vi "Weak AI Player.vi"(0 "Total Player number":i32, 1 "Current Player ID number":i32, 2 "queue output":refnum<queue>, 3 "queue input":refnum<queue>) -> ()   [LabVIEW 2021]
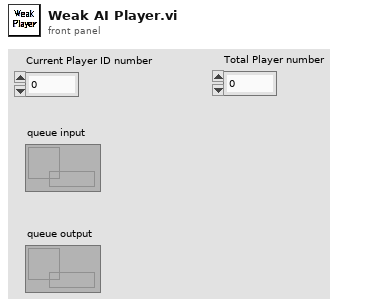
[diagram p1: front panel]
types:
  T1 = cluster{"X":dbl, "Y":dbl, "Object type":dbl, "Radius":dbl, "Width":dbl, "Height":dbl, "Theta":dbl, "HP":dbl, "R":dbl, "G":dbl, "B":dbl}[]
  T2 = cluster{"D1":dbl, "D2":dbl, "D3":dbl, "D4":dbl, "D5":dbl, "D6":dbl, "D7":dbl, "D8":dbl}
  T3 = cluster{"D1":bool, "D2":bool, "D3":bool, "D4":bool, "D5":bool, "D6":bool, "D7":bool, "D8":bool}
  T4 = cluster{"X":dbl, "Y":dbl, "Object type":dbl, "Radius":dbl, "Width":dbl, "Height":dbl, "Theta":dbl, "HP":dbl, "R":dbl, "G":dbl, "B":dbl}
  T5 = cluster{"Theta (toward that target)":dbl, "Distance (toward that target)":dbl, "Reachable":bool}
  T6 = cluster{dbl, dbl, "y":dbl, "y":dbl, "y":dbl, "y":dbl}
  T7 = cluster{dbl, dbl, "Theta (toward that target)":dbl, "f":dbl}
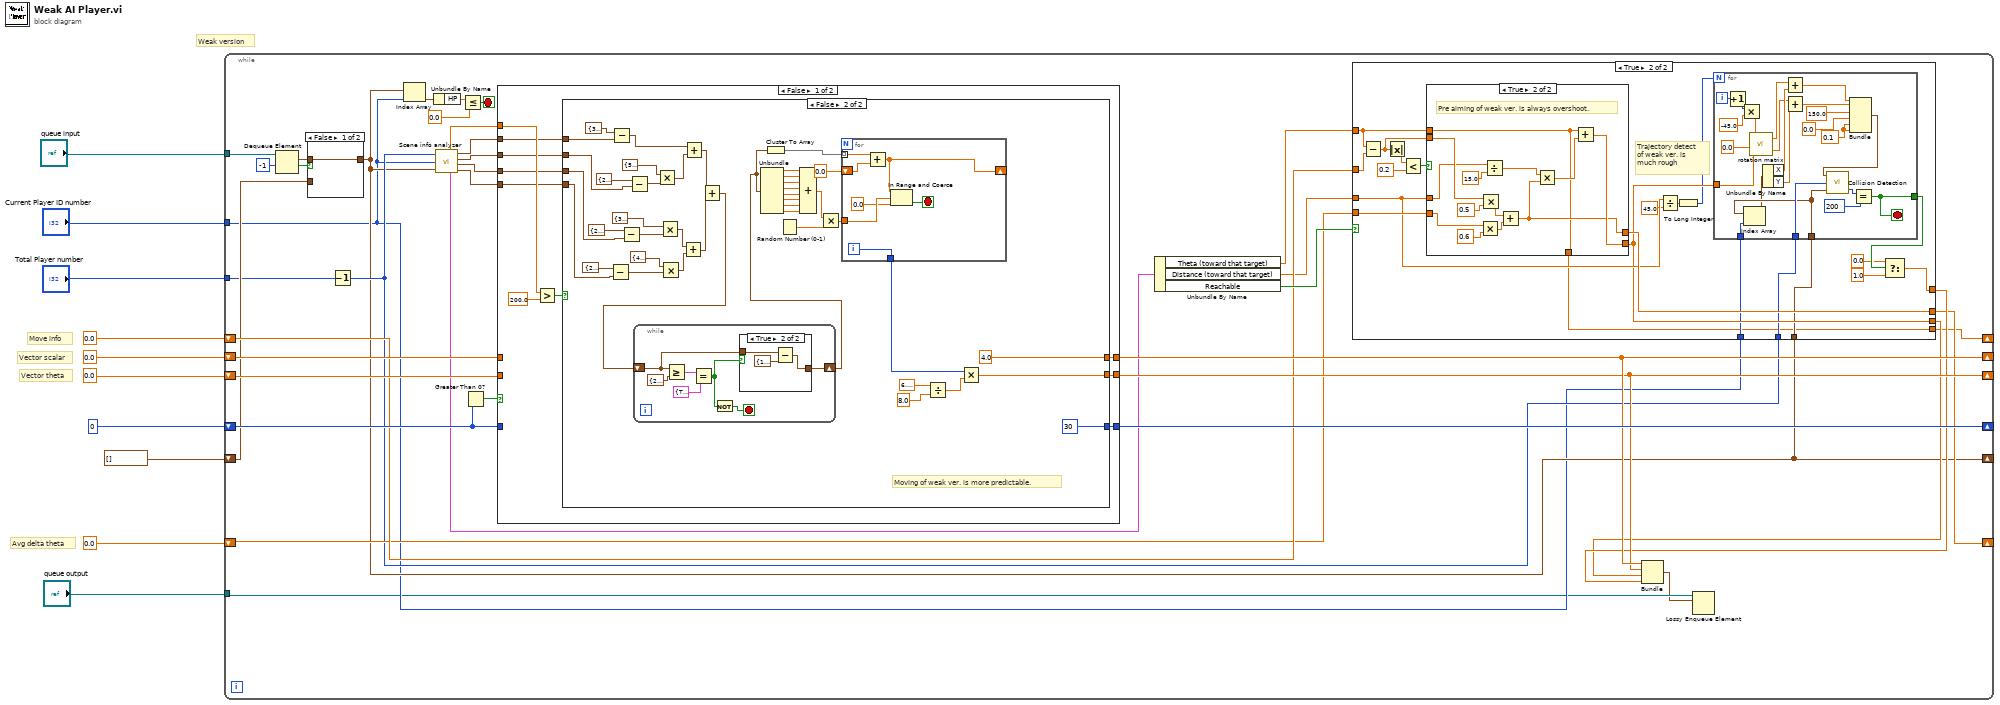
[diagram p0: block diagram]
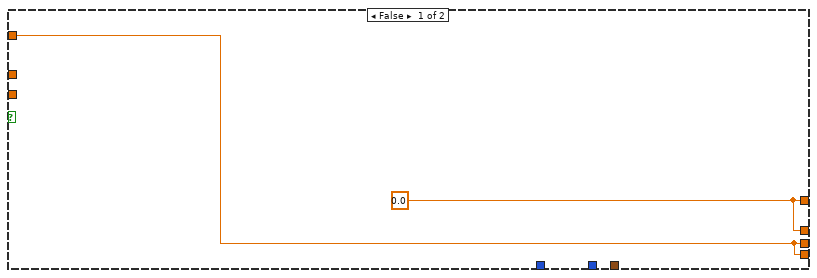
[diagram p3: hidden frame]
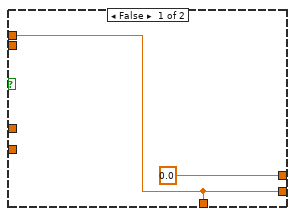
[diagram p4: hidden frame]
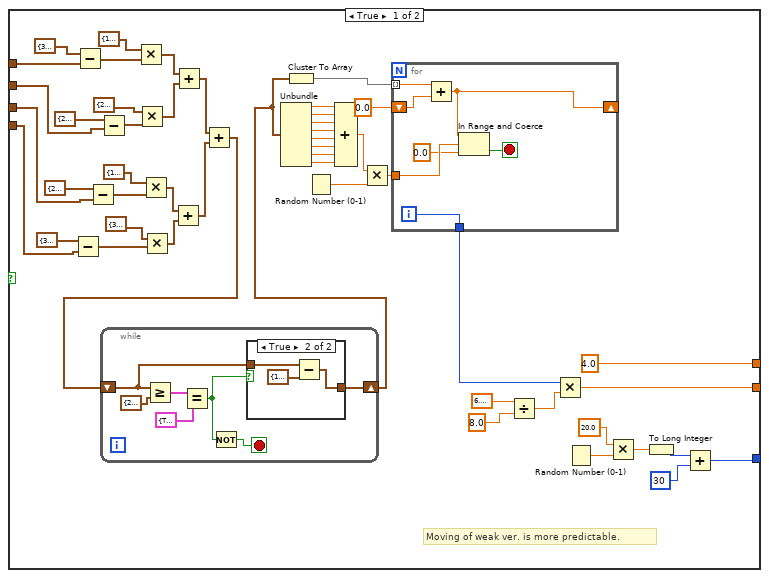
[diagram p5: hidden frame]
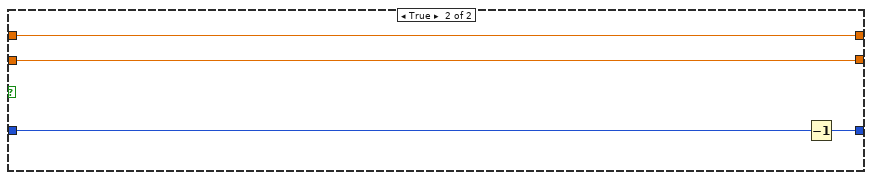
[diagram p8: hidden frame]
diagram:
  # "Weak version"
  # "Avg delta theta"
  # "Vector theta"
  # "Vector scalar"
  # "Move info"
  n1 = while {
    tunnel: "queue input" -> [w15]
    shift-right: [w47] -> _
    shift-left: 0 -> [w45]
    tunnel: "queue output" -> [w12]
    shift-right: [w21] -> _
    shift-left: 0.0 -> [w33]
    shift-right: [w37] -> _
    shift-left: 0.0 -> [w39]
    shift-right: [w36] -> _
    shift-left: 0.0 -> [w38]
    shift-right: [w27] -> _
    shift-left: 0.0 -> [w28]
    shift-right: [w20] -> _
    shift-left: T1 [] ("Map Entity Object Position") -> [w19]
    tunnel: "Current Player ID number" -> [w18]
    tunnel: "Total Player number" -> [w17]
    stop <- w23 stop-if-true
    n2 = Dequeue Element(queue=w15, timeout in ms (-1)=-1) -> (element=w16:T1, timed out?=w13:bool)  [unwired: 1 in, 2 out]
    n3 = case shown="False" w13 {
      tunnel: [w48 w49] -> w20
      tunnel: w16 -> [w48 _]
      tunnel: w19 -> [_ w49]
      frame False {
      }
      frame True {
      }
    }
    n4 = Decrement(x=w17) -> (x-1=w26:i32)
    n5 = Index Array(array=w20, index=w18) -> (element=w25:T4)
    n6 = Unbundle By Name(w25) -> ("HP"=w24:dbl)
    n7 = call "Scene info analyzer.vi"("Map Entity Object Position"=w20, "Current Player ID"=w18, "Max Player ID"=w26) -> ("Enemy on 8 directions"=w40:T2, "Closest valid target"=w35:T5, "Farther Bullets on 8 directions"=w41:T2, "Closer Bullets on 8 directions"=w42:T2, "Current Player HP"=w44:dbl, "Object on 8 directions"=w43:T2)
    n8 = Less Or Equal?(x=w24, y=0.0) -> (x <= y?=w23:bool)
    n9 = Greater Than 0?(x=w45) -> (x > 0?=w46:bool)
    n10 = case shown="False" w46 {
      tunnel: [w111 w250] -> w47
      tunnel: w45 -> [_ w251]
      tunnel: w44 -> [w118 _]
      tunnel: w43 -> [w117 _]
      tunnel: w42 -> [w116 _]
      tunnel: w41 -> [w115 _]
      tunnel: w40 -> [w114 _]
      tunnel: w39 -> [_ w249]
      tunnel: w38 -> [_ w248]
      tunnel: [w113 w248] -> w36
      tunnel: [w112 w249] -> w37
      frame False {
        n11 = Greater?(x=w118, y=200.0) -> (0:w120:bool)
        n12 = case shown="False" w120 {
          tunnel: w117 -> [w169 w229]
          tunnel: w116 -> [w167 w227]
          tunnel: w115 -> [w166 w226]
          tunnel: w114 -> [w165 w225]
          tunnel: [w134 w195] -> w113
          tunnel: [4.0 4.0] -> w112
          tunnel: [w132 30] -> w111
          frame True {
            # "Moving of weak ver. is more predictable."
            n13 = Subtract(x=T2 {"D1"=3.0, "D2"=3.0, "D3"=3.0, "D4"=3.0, "D5"=3.0, "D6"=3.0, "D7"=3.0, "D8"=3.0} ("Object on 8 directions"), y=w165) -> (x-y=w159:T2)
            n14 = Subtract(x=T2 {"D1"=3.0, "D2"=3.0, "D3"=3.0, "D4"=3.0, "D5"=3.0, "D6"=3.0, "D7"=3.0, "D8"=3.0} ("Object on 8 directions"), y=w169) -> (x-y=w124:T2)
            n15 = Subtract(x=T2 {"D1"=2.0, "D2"=2.0, "D3"=2.0, "D4"=2.0, "D5"=2.0, "D6"=2.0, "D7"=2.0, "D8"=2.0} ("Object on 8 directions"), y=w166) -> (x-y=w162:T2)
            n16 = Subtract(x=T2 {"D1"=2.0, "D2"=2.0, "D3"=2.0, "D4"=2.0, "D5"=2.0, "D6"=2.0, "D7"=2.0, "D8"=2.0} ("Object on 8 directions"), y=w167) -> (x-y=w164:T2)
            n17 = Multiply(x=T2 {"D1"=1.5, "D2"=1.5, "D3"=1.5, "D4"=1.5, "D5"=1.5, "D6"=1.5, "D7"=1.5, "D8"=1.5} ("Object on 8 directions"), y=w124) -> (x*y=w125:T2)
            n18 = Multiply(x=T2 {"D1"=2.0, "D2"=2.0, "D3"=2.0, "D4"=2.0, "D5"=2.0, "D6"=2.0, "D7"=2.0, "D8"=2.0} ("Object on 8 directions"), y=w164) -> (x*y=w157:T2)
            n19 = Multiply(x=T2 {"D1"=1.5, "D2"=1.5, "D3"=1.5, "D4"=1.5, "D5"=1.5, "D6"=1.5, "D7"=1.5, "D8"=1.5} ("Object on 8 directions"), y=w162) -> (x*y=w156:T2)
            n20 = Multiply(x=T2 {"D1"=3.0, "D2"=3.0, "D3"=3.0, "D4"=3.0, "D5"=3.0, "D6"=3.0, "D7"=3.0, "D8"=3.0} ("Object on 8 directions"), y=w159) -> (x*y=w155:T2)
            n21 = Add(x=w156, y=w155) -> (x+y=w153:T2)
            n22 = Add(x=w125, y=w157) -> (x+y=w154:T2)
            n23 = Add(x=w154, y=w153) -> (x+y=w123:T2)
            n24 = while {
              shift-right: [w172] -> w122
              shift-left: w123 -> [w171]
              stop <- w173 stop-if-true
              n25 = Greater Or Equal?(x=w171, y=T2 {"D1"=2.0, "D2"=2.0, "D3"=2.0, "D4"=2.0, "D5"=2.0, "D6"=2.0, "D7"=2.0, "D8"=2.0} ("Object on 8 directions")) -> (x >= y?=w175:T3)
              n26 = Equal?(x=w175, y=T3 {"D1"=TRUE, "D2"=TRUE, "D3"=TRUE, "D4"=TRUE, "D5"=TRUE, "D6"=TRUE, "D7"=TRUE, "D8"=TRUE}) -> (x = y?=w170:bool)
              n27 = Not(x=w170) -> (.not. x?=w173:bool)
              n28 = case shown="True" w170 {
                tunnel: [w177 w179] -> w172
                tunnel: w171 -> [w177 w178]
                frame False {
                }
                frame True {
                  n29 = Subtract(x=w178, y=T2 {"D1"=1.0, "D2"=1.0, "D3"=1.0, "D4"=1.0, "D5"=1.0, "D6"=1.0, "D7"=1.0, "D8"=1.0} ("Object on 8 directions")) -> (x-y=w179:T2)
                }
              }
            }
            n30 = Unbundle(w122) -> ("D1"=w152:dbl, "D2"=w151:dbl, "D3"=w150:dbl, "D4"=w149:dbl, "D5"=w148:dbl, "D6"=w147:dbl, "D7"=w146:dbl, "D8"=w145:dbl)
            n31 = Cluster To Array(cluster=w122) -> (array=w142:dbl[])
            n32 = Random Number (0-1)() -> (number: 0 to 1=w144:dbl)
            n33 = Compound Arithmetic op=ADD(w152, w151, w150, w149, w148, w147, w146, w145) -> (w143:dbl)
            n34 = Multiply(x=w143, y=w144) -> (x*y=w140:dbl)
            n35 = for {
              tunnel: w142 -> [w186] mode=indexing
              shift-right: [w185] -> _
              shift-left: 0.0 -> [w187]
              tunnel: w140 -> [w184]
              tunnel: [w183] -> w136
              i -> [w183]
              stop <- w182 stop-if-true
              n36 = Add(x=w186, y=w187) -> (x+y=w185:dbl)
              n37 = In Range and Coerce(upper limit=w185, x=w184, lower limit=0.0) -> (In Range?=w182:bool)  [unwired: 1 out]
            }
            n38 = Divide(x=6.283185307179586, y=8.0) -> (x/y=w137:dbl)
            n39 = Multiply(x=w136, y=w137) -> (x*y=w134:dbl)
            n40 = Random Number (0-1)() -> (number: 0 to 1=w131:dbl)
            n41 = Multiply(x=20.0, y=w131) -> (x*y=w130:dbl)
            n42 = To Long Integer(number=w130) -> (32bit integer=w128:i32)
            n43 = Add(x=w128, y=30) -> (x+y=w132:i32)
          }
          frame False {
            # "Moving of weak ver. is more predictable."
            n44 = Subtract(x=T2 {"D1"=2.0, "D2"=2.0, "D3"=2.0, "D4"=2.0, "D5"=2.0, "D6"=2.0, "D7"=2.0, "D8"=2.0} ("Object on 8 directions"), y=w225) -> (x-y=w221:T2)
            n45 = Subtract(x=T2 {"D1"=3.0, "D2"=3.0, "D3"=3.0, "D4"=3.0, "D5"=3.0, "D6"=3.0, "D7"=3.0, "D8"=3.0} ("Object on 8 directions"), y=w229) -> (x-y=w219:T2)
            n46 = Subtract(x=T2 {"D1"=2.0, "D2"=2.0, "D3"=2.0, "D4"=2.0, "D5"=2.0, "D6"=2.0, "D7"=2.0, "D8"=2.0} ("Object on 8 directions"), y=w226) -> (x-y=w223:T2)
            n47 = Subtract(x=T2 {"D1"=2.0, "D2"=2.0, "D3"=2.0, "D4"=2.0, "D5"=2.0, "D6"=2.0, "D7"=2.0, "D8"=2.0} ("Object on 8 directions"), y=w227) -> (x-y=w224:T2)
            n48 = Multiply(x=T2 {"D1"=5.0, "D2"=5.0, "D3"=5.0, "D4"=5.0, "D5"=5.0, "D6"=5.0, "D7"=5.0, "D8"=5.0} ("Object on 8 directions"), y=w224) -> (x*y=w218:T2)
            n49 = Multiply(x=T2 {"D1"=3.0, "D2"=3.0, "D3"=3.0, "D4"=3.0, "D5"=3.0, "D6"=3.0, "D7"=3.0, "D8"=3.0} ("Object on 8 directions"), y=w223) -> (x*y=w217:T2)
            n50 = Multiply(x=T2 {"D1"=4.0, "D2"=4.0, "D3"=4.0, "D4"=4.0, "D5"=4.0, "D6"=4.0, "D7"=4.0, "D8"=4.0} ("Object on 8 directions"), y=w221) -> (x*y=w216:T2)
            n51 = Add(x=w217, y=w216) -> (x+y=w214:T2)
            n52 = Add(x=w219, y=w218) -> (x+y=w215:T2)
            n53 = Add(x=w215, y=w214) -> (x+y=w189:T2)
            n54 = while {
              shift-right: [w232] -> w190
              shift-left: w189 -> [w231]
              stop <- w233 stop-if-true
              n55 = Greater Or Equal?(x=w231, y=T2 {"D1"=2.0, "D2"=2.0, "D3"=2.0, "D4"=2.0, "D5"=2.0, "D6"=2.0, "D7"=2.0, "D8"=2.0} ("Object on 8 directions")) -> (x >= y?=w235:T3)
              n56 = Equal?(x=w235, y=T3 {"D1"=TRUE, "D2"=TRUE, "D3"=TRUE, "D4"=TRUE, "D5"=TRUE, "D6"=TRUE, "D7"=TRUE, "D8"=TRUE}) -> (x = y?=w230:bool)
              n57 = Not(x=w230) -> (.not. x?=w233:bool)
              n58 = case shown="True" w230 {
                tunnel: [w237 w239] -> w232
                tunnel: w231 -> [w237 w238]
                frame False {
                }
                frame True {
                  n59 = Subtract(x=w238, y=T2 {"D1"=1.0, "D2"=1.0, "D3"=1.0, "D4"=1.0, "D5"=1.0, "D6"=1.0, "D7"=1.0, "D8"=1.0} ("Object on 8 directions")) -> (x-y=w239:T2)
                }
              }
            }
            n60 = Unbundle(w190) -> ("D1"=w213:dbl, "D2"=w212:dbl, "D3"=w211:dbl, "D4"=w210:dbl, "D5"=w209:dbl, "D6"=w208:dbl, "D7"=w207:dbl, "D8"=w206:dbl)
            n61 = Cluster To Array(cluster=w190) -> (array=w203:dbl[])
            n62 = Random Number (0-1)() -> (number: 0 to 1=w205:dbl)
            n63 = Compound Arithmetic op=ADD(w213, w212, w211, w210, w209, w208, w207, w206) -> (w204:dbl)
            n64 = Multiply(x=w204, y=w205) -> (x*y=w201:dbl)
            n65 = for {
              tunnel: w203 -> [w246] mode=indexing
              shift-right: [w245] -> _
              shift-left: 0.0 -> [w247]
              tunnel: w201 -> [w244]
              tunnel: [w243] -> w197
              i -> [w243]
              stop <- w242 stop-if-true
              n66 = Add(x=w246, y=w247) -> (x+y=w245:dbl)
              n67 = In Range and Coerce(upper limit=w245, x=w244, lower limit=0.0) -> (In Range?=w242:bool)  [unwired: 1 out]
            }
            n68 = Divide(x=6.283185307179586, y=8.0) -> (x/y=w198:dbl)
            n69 = Multiply(x=w197, y=w198) -> (x*y=w195:dbl)
          }
        }
      }
      frame True {
        n70 = Decrement(x=w251) -> (x-1=w250:i32)
      }
    }
    n71 = Unbundle By Name(w35) -> ("Theta (toward that target)"=w30:dbl, "Distance (toward that target)"=w29:dbl, "Reachable"=w34:bool)
    n72 = case shown="True" w34 {
      tunnel: w33 -> [w50 w72]
      tunnel: [w50 w61] -> w31
      tunnel: [w51 w56] -> w32
      tunnel: w30 -> [_ w68]
      tunnel: w29 -> [_ w64]
      tunnel: w28 -> [_ w65]
      tunnel: [w51 w67] -> w27
      tunnel: w20 -> [_ w60]
      tunnel: w26 -> [_ w55]
      tunnel: w18 -> [_ w54]
      tunnel: [w50 w53] -> w21
      frame False {
        w51 = 0.0
      }
      frame True {
        # "Trajectory detect \nof weak ver. is \nmuch rough"
        n73 = Subtract(x=w68, y=w72) -> (x-y=w66:dbl)
        n74 = Absolute Value(x=w66) -> (abs(x)=w70:dbl)
        n75 = Less?(x=w70, y=0.2) -> (x < y?=w71:bool)
        n76 = case shown="True" w71 {
          tunnel: [w96 w106] -> w61
          tunnel: w68 -> [w96 w98]
          tunnel: [0.0 w101] -> w67
          tunnel: w65 -> [_ w104]
          tunnel: w66 -> [_ w105]
          tunnel: w64 -> [_ w102]
          tunnel: [w96 w98] -> w53
          frame False {
          }
          frame True {
            # "Pre aiming of weak ver. is always overshoot."
            n77 = Multiply(x=w104, y=0.6) -> (x*y=w110:dbl)
            n78 = Multiply(x=w105, y=0.5) -> (x*y=w107:dbl)
            n79 = Divide(x=w102, y=15.0) -> (x/y=w99:dbl)
            n80 = Add(x=w107, y=w110) -> (x+y=w101:dbl)
            n81 = Multiply(x=w99, y=w101) -> (x*y=w100:dbl)
            n82 = Add(x=w98, y=w100) -> (x+y=w106:dbl)
          }
        }
        n83 = Divide(x=w64, y=45.0) -> (x/y=w62:dbl)
        n84 = To Long Integer(number=w62) -> (32bit integer=w52:i32)
        n85 = for {
          N: w52 -> [_]
          tunnel: w61 -> [w95]
          tunnel: w60 -> [w85]
          tunnel: [w73] -> w59
          tunnel: w55 -> [w91]
          tunnel: w54 -> [w86]
          i -> [w89]
          stop <- w73 stop-if-true
          w83 = 0.1 ("y")
          n86 = Increment(x=w89) -> (x+1=w88:i32)
          n87 = Multiply(x=w88, y=-45.0) -> (x*y=w87:dbl)
          n88 = Index Array(array=w85, index=w86) -> (element=w84:T4)
          n89 = call "rotation matrix.vi"("angle"=w95, "y"=0.0, "x"=w87) -> ("new y"=w77:dbl, "new x"=w76:dbl)
          n90 = Unbundle By Name(w84) -> ("X"=w78:dbl, "Y"=w79:dbl)
          n91 = Add(x=w76, y=w78) -> (x+y=w75:dbl)
          n92 = Add(x=w77, y=w79) -> (x+y=w74:dbl)
          n93 = Bundle(w75, w74, "y"=150.0, "y"=0.0, "y"=w83, "y"=w83) -> (w82:T6)  [unwired: 1 in]
          n94 = call "Collision Detection.vi"("Map Entity Objects Positions"=w85, "Max Player ID number"=w91, "Moving Object"=w82) -> ("Bullet hit Player No."=w93:i32)  [unwired: 1 out]
          n95 = Equal?(x=w93, y=200) -> (x = y?=w73:bool)
        }
        n96 = Select(t=0.0, s=w59, f=1.0) -> (s? t:f=w56:dbl)
      }
    }
    n97 = Bundle(w37, w36, "Theta (toward that target)"=w31, "f"=w32) -> (w11:T7)  [unwired: 1 in]
    n98 = Lossy Enqueue Element(queue=w12, element=w11) -> ()  [unwired: 1 in, 4 out]
  }
